vi "Wait for Msg Complete.vi"(11 "Queue in":T1) -> (3 "Queue out":T1)   [LabVIEW 2019]
uses:
  <vilib>/NI/AMC/Message Queue.ctl
  <vilib>/NI/AMC/Message.ctl
  <vilib>/NI/Tools/Keyed Array/KeyedArray.ctl
  <vilib>/NI/AMC/AMC.lvlib
  <vilib>/NI/Tools/Keyed Array/Tools_KeyedArray.lvlib
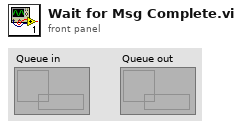
[diagram p1: front panel]
types:
  T1 = typedef "AMC.lvlib/Message Queue.ctl" = refnum<queue>
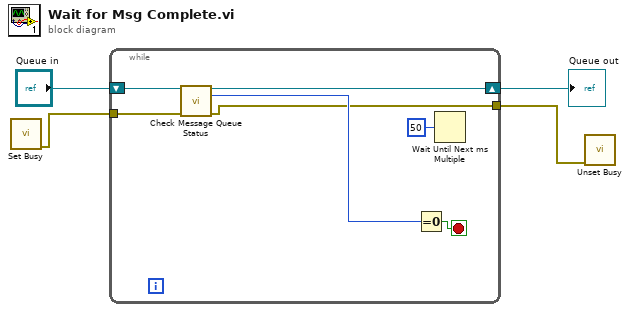
[diagram p0: block diagram]
diagram:
  n1 = call <vilib>:"Set Busy.vi"() -> ("error out"=w2:errorcluster)  [unwired: 10 in, 1 out]
  n2 = while {
    shift-right: [w11] -> w3
    shift-left: "Queue in" -> [w10]
    tunnel: w2 -> [w6]
    tunnel: [w5] -> w1
    stop <- w8 stop-if-true
    n3 = call <vilib>:"Check Message Queue Status.vi"("message queue in"=w10, "error in"=w6) -> ("message queue out"=w11:T1, "# elements in queue"=w9:i32, "error out"=w5:errorcluster)  [unwired: 9 in, 2 out]
    n4 = Equal To 0?(x=w9) -> (x = 0?=w8:bool)
    n5 = Wait Until Next ms Multiple(millisecond multiple=u32 50) -> ()  [unwired: 1 out]
  }
  "Queue out" <- w3
  n6 = call <vilib>:"Unset Busy.vi"("error in (no error)"=w1) -> ()  [unwired: 10 in, 1 out]
